vi "Start Video-reinitiate imaq.vi"(5 "Offset":cluster{"Ch1":u8, "Ch2":u8}, 7 "Gain(dB)":cluster{"Ch1":dbl, "Ch2":dbl}, 8 "error in":errorcluster, 9 "Camera Fr":u16, 10 "Trigger Type":enum16{"Internal", "External"}(ring)=enum."External", 11 "Region of interest":i32[](array[numeric])) -> (0 "error out":errorcluster, 1 "Frame Buffers Out":T1[](array[typedef]), 3 "IMAQ Session Out":refnum<k11>)   [LabVIEW 2013]
uses:
  <vilib>/vision/Image Controls.llb/IMAQ Image.ctl
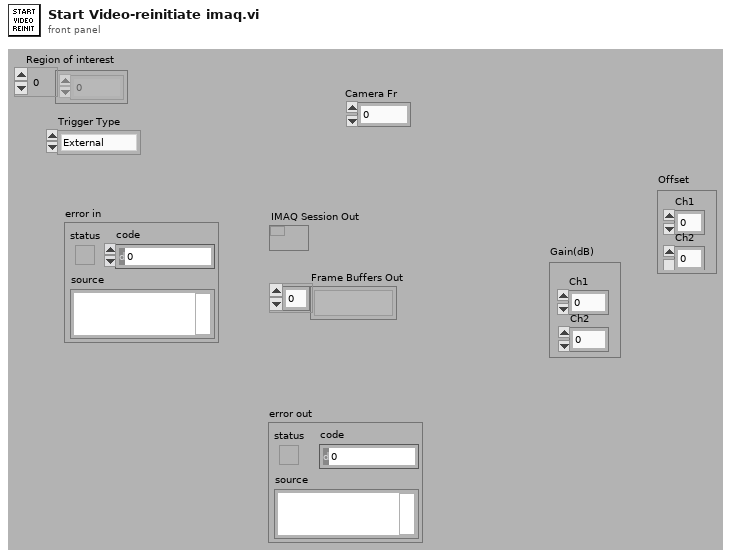
[diagram p1: front panel]
types:
  T1 = typedef "IMAQ Image.ctl" = refnum<image>
  T2 = typedef "Image Type" = u32
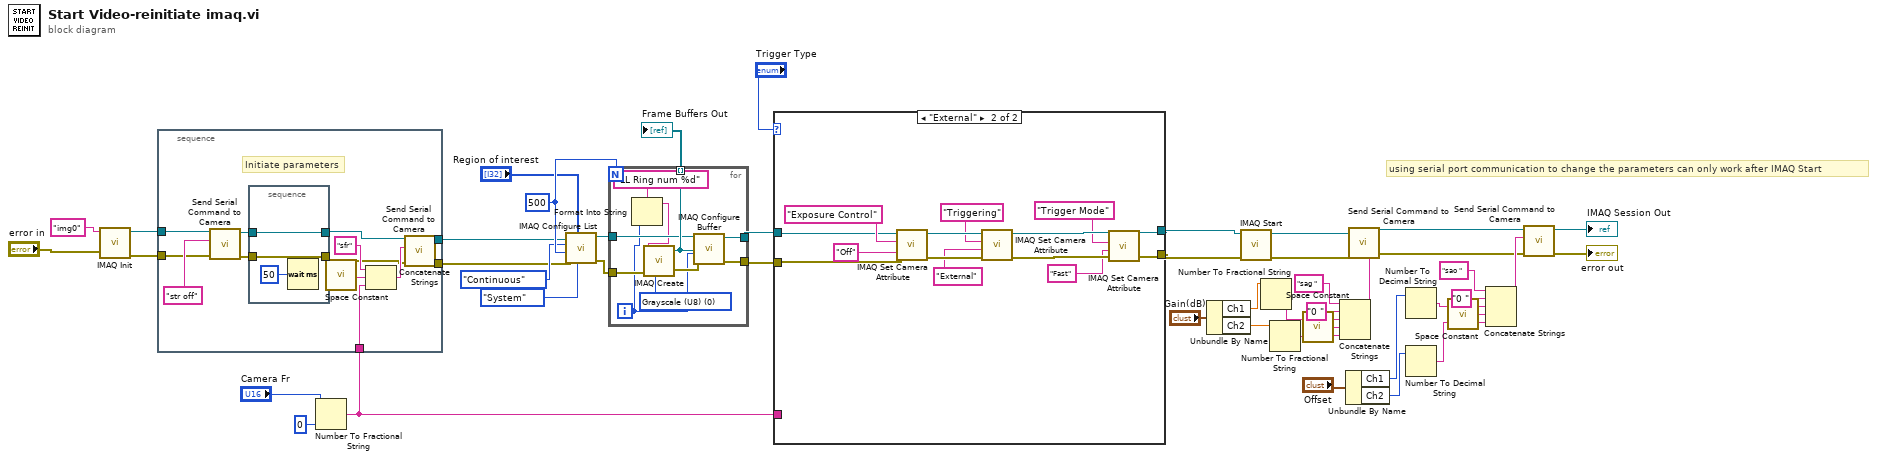
[diagram p0: block diagram]
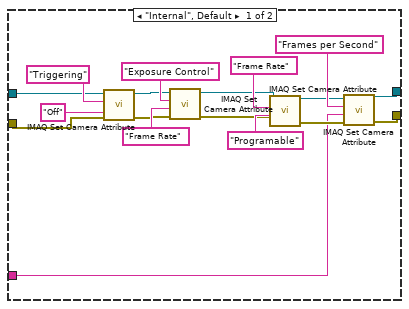
[diagram p2: hidden frame]
diagram:
  w45 = 500 ("Number of buffers")
  # "using serial port communication to change the parameters can only work after IMAQ Start"
  n1 = call <vilib>:"IMAQ Init.vi"("error in (no error)"="error in", "Interface Name"="img0") -> ("error out"=w34:errorcluster, "IMAQ Session Out"=w35:refnum<k11>)  [unwired: 8 in]
  n2 = Number To Fractional String(number="Camera Fr", precision (6)=i16 0) -> (F-format string=w30:string)  [unwired: 2 in]
  n3 = stacked-sequence {
    tunnel: w35 -> [w50]
    tunnel: w34 -> [w49]
    tunnel: [w48] -> w33
    tunnel: [w47] -> w32
    tunnel: w30 -> [w46]
    frame #0 {
      # "Initiate parameters"
      n4 = call "Send Serial Command to Camera.vi"("error in (no error)"=w49, "String to write"="str off", "IMAQ Session In"=w50) -> ("error out"=w52:errorcluster, "IMAQ Session Out"=w54:refnum<k11>)  [unwired: 5 in, 2 out]
      n5 = stacked-sequence {
        tunnel: w54 -> [w61]
        tunnel: [w61] -> w53
        tunnel: w52 -> [w60]
        tunnel: [w60] -> w51
        frame #0 {
          n6 = Wait (ms)(milliseconds to wait=u32 50) -> ()  [unwired: 1 out]
        }
      }
      n7 = call <vilib>:"Space Constant.vi"() -> ("String"=w56:string)
      n8 = Concatenate Strings("sfr" ("string"), w56, w46) -> (w55:string)
      n9 = call "Send Serial Command to Camera.vi"("error in (no error)"=w51, "String to write"=w55, "IMAQ Session In"=w53) -> ("error out"=w47:errorcluster, "IMAQ Session Out"=w48:refnum<k11>)  [unwired: 5 in, 2 out]
    }
  }
  n10 = call <vilib>:"IMAQ Configure List.vi"("Memory Location"=enum16{"System", "Onboard"}."System", "Region of interest"="Region of interest", "error in (no error)"=w32, "Number of buffers"=w45, "Continuous?"=enum16{"One-Shot", "Continuous"}."Continuous" ("Continuous ?"), "IMAQ Session In"=w33) -> ("error out"=w38:errorcluster, "IMAQ Session Out"=w39:refnum<k11>)  [unwired: 4 in]
  n11 = for {
    N: w45 -> [_]
    tunnel: [w71] -> w37
    tunnel: [w63] -> w36
    tunnel: w38 -> [w70]
    tunnel: w39 -> [w67]
    tunnel: [w68] -> w43 mode=indexing
    i -> [w64]
    w62 = T2 0 items=["Grayscale (U8)", "Grayscale (I16)", "Grayscale (SGL)", "Complex (CSG)", "RGB (U32)", "HSL (U32)", "RGB (U64)"] ("Image Type")
    n12 = Format Into String(format string="LL Ring num %d", w64) -> (resulting string=w66:string)  [unwired: 2 in, 1 out]
    n13 = call "IMAQ Create"("Image Name"=w66, "Image Type"=w62, "error in (no error)"=w70) -> ("New Image"=w68:T1, "error out"=w69:errorcluster)  [unwired: 2 in]
    n14 = call <vilib>:"IMAQ Configure Buffer.vi"("error in (no error)"=w69, "Buffer Number"=w64, "Image In"=w68, "IMAQ Session In"=w67) -> ("error out"=w63:errorcluster, "IMAQ Session Out"=w71:refnum<k11>)  [unwired: 6 in]
  }
  "Frame Buffers Out" <- w43
  n15 = case shown="\"External\"" "Trigger Type" {
    tunnel: w37 -> [w76 w93]
    tunnel: w36 -> [w75 w92]
    tunnel: w30 -> [w74 _]
    tunnel: [w73 w90] -> w29
    tunnel: [w72 w91] -> w28
    frame "Internal", Default {
      n16 = call <vilib>:"IMAQ Set Camera Attribute.vi"("error in (no error)"=w75, "Attribute Value"="Off", "Camera Attribute"="Triggering", "IMAQ Session In"=w76) -> ("error out"=w81:errorcluster, "IMAQ Session Out"=w83:refnum<k11>)  [unwired: 4 in]
      n17 = call <vilib>:"IMAQ Set Camera Attribute.vi"("error in (no error)"=w81, "Attribute Value"="Frame Rate", "Camera Attribute"="Exposure Control", "IMAQ Session In"=w83) -> ("error out"=w82:errorcluster, "IMAQ Session Out"=w84:refnum<k11>)  [unwired: 4 in]
      n18 = call <vilib>:"IMAQ Set Camera Attribute.vi"("error in (no error)"=w82, "Attribute Value"="Programable", "Camera Attribute"="Frame Rate", "IMAQ Session In"=w84) -> ("error out"=w80:errorcluster, "IMAQ Session Out"=w79:refnum<k11>)  [unwired: 4 in]
      n19 = call <vilib>:"IMAQ Set Camera Attribute.vi"("error in (no error)"=w80, "Attribute Value"=w74, "Camera Attribute"="Frames per Second", "IMAQ Session In"=w79) -> ("error out"=w72:errorcluster, "IMAQ Session Out"=w73:refnum<k11>)  [unwired: 4 in]
    }
    frame "External" {
      n20 = call <vilib>:"IMAQ Set Camera Attribute.vi"("error in (no error)"=w92, "Attribute Value"="Off", "Camera Attribute"="Exposure Control", "IMAQ Session In"=w93) -> ("error out"=w101:errorcluster, "IMAQ Session Out"=w99:refnum<k11>)  [unwired: 4 in]
      n21 = call <vilib>:"IMAQ Set Camera Attribute.vi"("error in (no error)"=w101, "Attribute Value"="External", "Camera Attribute"="Triggering", "IMAQ Session In"=w99) -> ("error out"=w100:errorcluster, "IMAQ Session Out"=w98:refnum<k11>)  [unwired: 4 in]
      n22 = call <vilib>:"IMAQ Set Camera Attribute.vi"("error in (no error)"=w100, "Attribute Value"="Fast", "Camera Attribute"="Trigger Mode", "IMAQ Session In"=w98) -> ("error out"=w91:errorcluster, "IMAQ Session Out"=w90:refnum<k11>)  [unwired: 4 in]
    }
  }
  n23 = Unbundle By Name("Gain(dB)") -> ("Ch1"=w17:dbl, "Ch2"=w16:dbl)
  n24 = call <vilib>:"IMAQ Start.vi"("error in (no error)"=w28, "IMAQ Session In"=w29) -> ("error out"=w18:errorcluster, "IMAQ Session Out"=w19:refnum<k11>)  [unwired: 8 in]
  n25 = Number To Fractional String(number=w17) -> (F-format string=w21:string)  [unwired: 3 in]
  n26 = Number To Fractional String(number=w16) -> (F-format string=w23:string)  [unwired: 3 in]
  n27 = call <vilib>:"Space Constant.vi"() -> ("String"=w22:string)
  n28 = Concatenate Strings("sag " ("String to write"), "0 " ("string"), w21, w22, w23) -> (w20:string)
  n29 = Unbundle By Name("Offset") -> ("Ch1"=w7:u8, "Ch2"=w6:u8)
  n30 = call "Send Serial Command to Camera.vi"("error in (no error)"=w18, "String to write"=w20, "IMAQ Session In"=w19) -> ("error out"=w8:errorcluster, "IMAQ Session Out"=w9:refnum<k11>)  [unwired: 5 in, 2 out]
  n31 = Number To Decimal String(number=w7) -> (decimal integer string=w11:string)  [unwired: 1 in]
  n32 = Number To Decimal String(number=w6) -> (decimal integer string=w10:string)  [unwired: 1 in]
  n33 = call <vilib>:"Space Constant.vi"() -> ("String"=w13:string)
  n34 = Concatenate Strings("sao " ("String to write"), "0 " ("string"), w11, w13, w10) -> (w12:string)
  n35 = call "Send Serial Command to Camera.vi"("error in (no error)"=w8, "String to write"=w12, "IMAQ Session In"=w9) -> ("error out"=→"error out":errorcluster, "IMAQ Session Out"=→"IMAQ Session Out":refnum<k11>)  [unwired: 5 in, 2 out]
